vi "Self-Test.vi"(8 "error in (no error)":errorcluster, 11 "VISA resource name":refnum<visa-resource-name>) -> (0 "error out":errorcluster, 1 "Self-Test Response":string, 2 "Self-Test Error":i32, 3 "VISA resource name out":refnum<visa-resource-name>)   [LabVIEW 2014, in "Associated Research SC6540.lvlib"]
doc: "Perform a self-test and returns the results. A string contains the instruments response, there is no Self-Test Error number returned by this VI."
uses:
  <instrlib>/Associated Research SC6540/Associated Research SC6540.lvlib
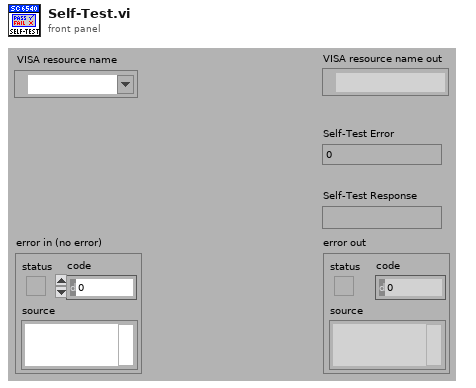
[diagram p1: front panel]
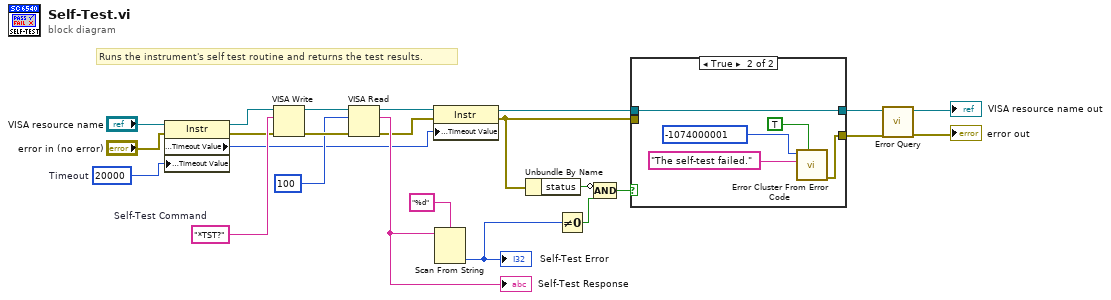
[diagram p0: block diagram]
diagram:
  w18 = u32 20000  # Timeout
  w19 = "*TST?"  # Self-Test Command
  # "Runs the instrument's self test routine and returns the test results."
  n1 = property class="Instr"(reference="VISA resource name", error in="error in (no error)", "General Settings:Timeout Value"=w18) -> (reference out=w15:refnum<visa-resource-name>, error out=w14:errorcluster, "General Settings:Timeout Value"=w11:u32)
  n2 = VISA Write(VISA resource name=w15, write buffer=w19, error in (no error)=w14) -> (VISA resource name out=w24:refnum<visa-resource-name>, error out=w22:errorcluster)  [unwired: 1 out]
  n3 = VISA Read(VISA resource name=w24, byte count=u32 100, error in (no error)=w22) -> (VISA resource name out=w13:refnum<visa-resource-name>, read buffer=w21:string, error out=w12:errorcluster)  [unwired: 1 out]
  "Self-Test Response" <- w21
  n4 = property class="Instr"(reference=w13, error in=w12, "General Settings:Timeout Value"=w11) -> (reference out=w5:refnum<visa-resource-name>, error out=w6:errorcluster)
  n5 = Scan From String(format string="%d" ("Format String"), input string=w21) -> (output 1=w7:i32)  [unwired: 3 in, 3 out]
  "Self-Test Error" <- w7
  n6 = Unbundle By Name(w6) -> ("status"=w9:bool)
  n7 = Not Equal To 0?(x=w7) -> (x != 0?=w10:bool)
  n8 = Compound Arithmetic op=AND(invert w9, w10) -> (w8:bool)
  n9 = case shown="True" w8 {
    tunnel: w5 -> [w26 w31]
    tunnel: w6 -> [w25 _]
    tunnel: [w25 w27] -> w2
    tunnel: [w26 w31] -> w4
    frame False {
    }
    frame True {
      n10 = call <vilib>:"Error Cluster From Error Code.vi"("show call chain? (False)"=TRUE, "error message (\"\")"="The self-test failed." ("Source (VI Name)"), "error code (0)"=-1074000001 ("Code")) -> ("error out"=w27:errorcluster)  [unwired: 6 in]
    }
  }
  n11 = call <instrlib>:"Error Query.vi"("error in (no error)"=w2, "VISA resource name"=w4) -> ("error out"=→"error out":errorcluster, "VISA resource name out"=→"VISA resource name out":refnum<visa-resource-name>)  [unwired: 6 in, 2 out]
